vi "ASIC_Selecor canal Sumador.vi"(7 "Espera acceso USB":u32=10, 8 "error in":errorcluster, 9 "Sumador":u8, 10 "Canal":u8, 11 "ftHandle_in":u32) -> (0 "error out":errorcluster, 2 "Reg 101-100":u32, 3 "ftHandle_out":u32)   [LabVIEW 2019]
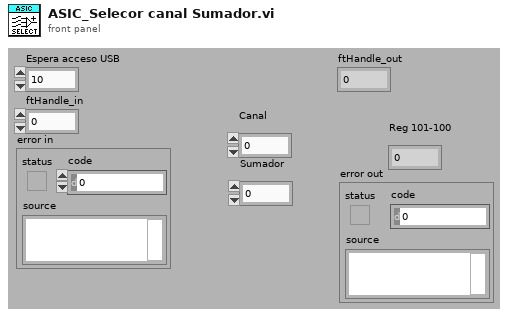
[diagram p1: front panel]
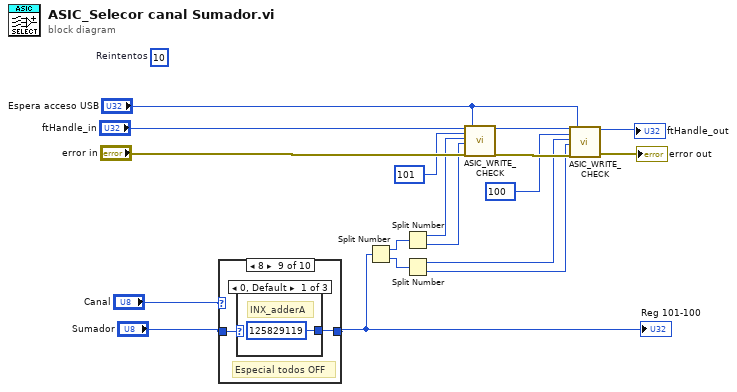
[diagram p0: block diagram]
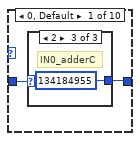
[diagram p2: hidden frame]
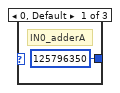
[diagram p3: hidden frame]
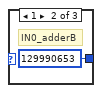
[diagram p4: hidden frame]
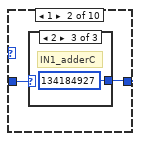
[diagram p5: hidden frame]
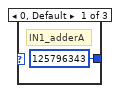
[diagram p6: hidden frame]
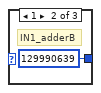
[diagram p7: hidden frame]
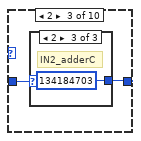
[diagram p8: hidden frame]
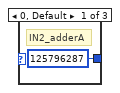
[diagram p9: hidden frame]
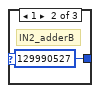
[diagram p10: hidden frame]
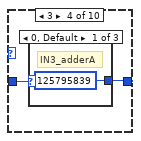
[diagram p11: hidden frame]
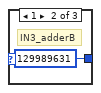
[diagram p12: hidden frame]
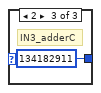
[diagram p13: hidden frame]
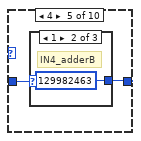
[diagram p14: hidden frame]
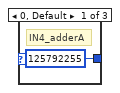
[diagram p15: hidden frame]
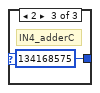
[diagram p16: hidden frame]
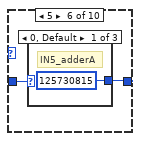
[diagram p17: hidden frame]
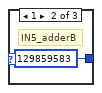
[diagram p18: hidden frame]
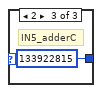
[diagram p19: hidden frame]
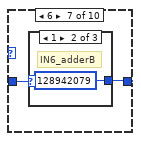
[diagram p20: hidden frame]
diagram:
  (unwired) 10  # Reintentos
  n1 = case shown="8" "Canal" {
    tunnel: "Sumador" -> [w20 w25 w30 w35 w40 w45 w50 w55 w60 w65]
    tunnel: [w19 w24 w29 w34 w39 w44 w49 w54 w59 w64] -> w14
    frame 0, Default {
      n2 = case shown="2" w20 {
        tunnel: [u32 125796350 ("Threshold Inicial N") u32 129990653 ("Threshold Inicial N") u32 134184955 ("Threshold Inicial N")] -> w19
        frame 0, Default {
          # "IN0_adderA"
        }
        frame 1 {
          # "IN0_adderB"
        }
        frame 2 {
          # "IN0_adderC"
        }
      }
    }
    frame 1 {
      n3 = case shown="2" w25 {
        tunnel: [u32 125796343 ("Threshold Inicial N") u32 129990639 ("Threshold Inicial N") u32 134184927 ("Threshold Inicial N")] -> w24
        frame 0, Default {
          # "IN1_adderA"
        }
        frame 1 {
          # "IN1_adderB"
        }
        frame 2 {
          # "IN1_adderC"
        }
      }
    }
    frame 2 {
      n4 = case shown="2" w30 {
        tunnel: [u32 125796287 ("Threshold Inicial N") u32 129990527 ("Threshold Inicial N") u32 134184703 ("Threshold Inicial N")] -> w29
        frame 0, Default {
          # "IN2_adderA"
        }
        frame 1 {
          # "IN2_adderB"
        }
        frame 2 {
          # "IN2_adderC"
        }
      }
    }
    frame 3 {
      n5 = case shown="0, Default" w35 {
        tunnel: [u32 125795839 ("Threshold Inicial N") u32 129989631 ("Threshold Inicial N") u32 134182911 ("Threshold Inicial N")] -> w34
        frame 0, Default {
          # "IN3_adderA"
        }
        frame 1 {
          # "IN3_adderB"
        }
        frame 2 {
          # "IN3_adderC"
        }
      }
    }
    frame 4 {
      n6 = case shown="1" w40 {
        tunnel: [u32 125792255 ("Threshold Inicial N") u32 129982463 ("Threshold Inicial N") u32 134168575 ("Threshold Inicial N")] -> w39
        frame 0, Default {
          # "IN4_adderA"
        }
        frame 1 {
          # "IN4_adderB"
        }
        frame 2 {
          # "IN4_adderC"
        }
      }
    }
    frame 5 {
      n7 = case shown="0, Default" w45 {
        tunnel: [u32 125730815 ("Threshold Inicial N") u32 129859583 ("Threshold Inicial N") u32 133922815 ("Threshold Inicial N")] -> w44
        frame 0, Default {
          # "IN5_adderA"
        }
        frame 1 {
          # "IN5_adderB"
        }
        frame 2 {
          # "IN5_adderC"
        }
      }
    }
    frame 6 {
      n8 = case shown="1" w50 {
        tunnel: [u32 125272063 ("Threshold Inicial N") u32 128942079 ("Threshold Inicial N") u32 132087807 ("Threshold Inicial N")] -> w49
        frame 0, Default {
          # "IN6_adderA"
        }
        frame 1 {
          # "IN6_adderB"
        }
        frame 2 {
          # "IN6_adderC"
        }
      }
    }
    frame 7 {
      n9 = case shown="0, Default" w55 {
        tunnel: [u32 125201846 ("Threshold Inicial N") u32 128801645 ("Threshold Inicial N") u32 131806939 ("Threshold Inicial N")] -> w54
        frame 0, Default {
          # "INX_adderA"
        }
        frame 1 {
          # "INX_adderB"
        }
        frame 2 {
          # "INX_adderC"
        }
      }
    }
    frame 8 {
      # "Especial todos OFF"
      n10 = case shown="0, Default" w60 {
        tunnel: [u32 125829119 ("Threshold Inicial N") u32 130023423 ("Threshold Inicial N") u32 134217727 ("Threshold Inicial N")] -> w59
        frame 0, Default {
          # "INX_adderA"
        }
        frame 1 {
          # "INX_adderB"
        }
        frame 2 {
          # "INX_adderC"
        }
      }
    }
    frame 9 {
      # "Especial todos On"
      n11 = case shown="0, Default" w65 {
        tunnel: [u32 121634816 ("Threshold Inicial N") u32 125829120 ("Threshold Inicial N") u32 130023424 ("Threshold Inicial N")] -> w64
        frame 0, Default {
          # "INX_adderA"
        }
        frame 1 {
          # "INX_adderB"
        }
        frame 2 {
          # "INX_adderC"
        }
      }
    }
  }
  "Reg 101-100" <- w14
  n12 = Split Number(x=w14) -> (hi(x)=w4:u16, lo(x)=w3:u16)
  n13 = Split Number(x=w4) -> (hi(x)=w10:u8, lo(x)=w9:u8)
  n14 = Split Number(x=w3) -> (hi(x)=w8:u8, lo(x)=w7:u8)
  n15 = call "ASIC_WRITE_CHECK.vi"("ftHandle_in"="ftHandle_in", "Direccion Registro Asic"=u8 101, "Byte Alto"=w10, "Byte Bajo"=w9, "error in"="error in", "Espera acceso USB 2"="Espera acceso USB") -> ("ftHandle_out"=w12:u32, "error out"=w11:errorcluster)  [unwired: 11 in, 1 out]
  n16 = call "ASIC_WRITE_CHECK.vi"("ftHandle_in"=w12, "Direccion Registro Asic"=u8 100, "Byte Alto"=w8, "Byte Bajo"=w7, "error in"=w11, "Espera acceso USB 2"="Espera acceso USB") -> ("ftHandle_out"=→"ftHandle_out":u32, "error out"=→"error out":errorcluster)  [unwired: 11 in, 1 out]
